vi "Combustion Setup 1.vi"() -> ()   [LabVIEW 2018]
doc: "Simplified example program for initializing the COM port, determining the data frame of an Alicat, acquiring the data of the same Alicat, and writing a setpoint to the same device. \n\nThis is a slightly more feature rich version of the Alicat Simplified Driver Example, and contains an example of a method for easily implementing fast setpoint writes."
panel:
  in  "Stopping Flow Rate (Top)":dbl format="%_4g"
  in  "Initial Flow Rate (Top)":dbl format="%_4g"
  in  "Top COM Port Settings (always Unit ID = B; methane)":T1={"Unit ID"="A", "Baud Rate"=enum."19200", "VISA Sesssion In"="COM1"}
  in  "Stopping Flow Rate (Bottom)":dbl format="%_4g"
  in  "Stop Running Button":bool
  in  "Initial Flow Rate (Bottom)":dbl format="%_4g"
  in  "Bottom COM Port Settings (always Unit ID = A; oxygen)":T1={"Unit ID"="A", "Baud Rate"=enum."19200", "VISA Sesssion In"="COM1"}
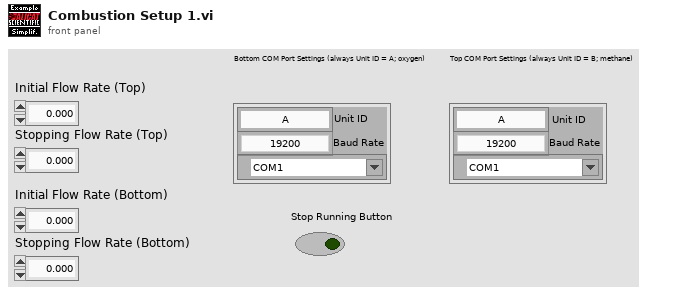
[diagram p1: front panel]
types:
  T1 = cluster{"Unit ID":string, "Baud Rate":enum8{"2400", "9600", "19200", "38400", "57600", "115200", "Unknown"}, "VISA Sesssion In":refnum<visa-resource-name>}
  T2 = cluster{"Absolute Pressure":bool, "Gauge/Diff. Pressure":bool, "Barometric Pressure":bool, "Temperature":bool, "Volumetric":bool, "Mass":bool, "Setpoint":bool, "Valve Drive":bool, "Totalizer":bool, "Totalizer Timer":bool, "Totalizer Average Flow":bool, "Totalizer Peak Flow":bool, "Gas Selected":bool, "Tot. Timer Format":u16}
  T3 = cluster{"Controller Full Scale":dbl, "Controller Select":u16, "Control Range":enum16{"Normal", "Inverted", "Bidirectional", "Unknown"}}
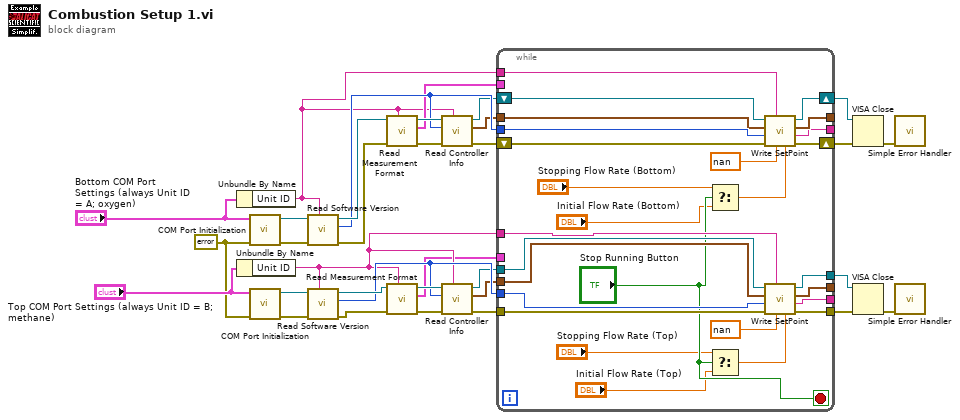
[diagram p0: block diagram]
diagram:
  w1 = errorcluster {"status"=FALSE, "code"=0, "source"=""} ("error in (no error)")
  n1 = Unbundle By Name("Bottom COM Port Settings (always Unit ID = A; oxygen)") -> ("Unit ID"=w6:string)
  n2 = Unbundle By Name("Top COM Port Settings (always Unit ID = B; methane)") -> ("Unit ID"=w17:string)
  n3 = call "COM Port Initialization.vi"("error in (no error)"=w1, "Communication Settings"="Bottom COM Port Settings (always Unit ID = A; oxygen)") -> ("error out"=w4:errorcluster, "VISA Session Out"=w3:refnum<visa-resource-name>)  [unwired: 8 in]
  n4 = call "COM Port Initialization.vi"("error in (no error)"=w1, "Communication Settings"="Top COM Port Settings (always Unit ID = B; methane)") -> ("error out"=w8:errorcluster, "VISA Session Out"=w9:refnum<visa-resource-name>)  [unwired: 8 in]
  n5 = call "Read Software Version.vi"("Unit ID (A)"=w6, "error in"=w4, "VISA Session In"=w3) -> ("error out"=w31:errorcluster, "Software Version"=w29:u8, "VISA Session Out"=w30:refnum<visa-resource-name>)  [unwired: 6 in]
  n6 = call "Read Software Version.vi"("Unit ID (A)"=w17, "error in"=w8, "VISA Session In"=w9) -> ("error out"=w22:errorcluster, "Software Version"=w20:u8, "VISA Session Out"=w21:refnum<visa-resource-name>)  [unwired: 6 in]
  n7 = call "Read Measurement Format.vi"("Unit ID (A)"=w6, "error in"=w31, "VISA Session In"=w30) -> ("error out"=w33:errorcluster, "Data Frame Format"=w7:T2, "VISA Session Out"=w32:refnum<visa-resource-name>)  [unwired: 6 in]
  n8 = call "Read Measurement Format.vi"("Unit ID (A)"=w17, "error in"=w22, "VISA Session In"=w21) -> ("error out"=w24:errorcluster, "Data Frame Format"=w5:T2, "VISA Session Out"=w23:refnum<visa-resource-name>)  [unwired: 6 in]
  n9 = call "Read Controller Info.vi"("Unit ID (A)"=w6, "error in"=w33, "Software Version"=w29, "VISA Session In"=w32) -> ("error out"=w28:errorcluster, "Controller Info out"=w27:T3, "VISA Session Out"=w26:refnum<visa-resource-name>)  [unwired: 4 in, 1 out]
  n10 = call "Read Controller Info.vi"("Unit ID (A)"=w17, "error in"=w24, "Software Version"=w20, "VISA Session In"=w23) -> ("error out"=w19:errorcluster, "Controller Info out"=w18:T3, "VISA Session Out"=w16:refnum<visa-resource-name>)  [unwired: 4 in, 1 out]
  n11 = while {
    tunnel: w29 -> [w60]
    tunnel: w27 -> [w58]
    tunnel: w20 -> [w54]
    tunnel: w19 -> [w53]
    tunnel: w18 -> [w52]
    tunnel: w17 -> [w51]
    tunnel: w16 -> [w49]
    shift-right: [w46] -> w14
    shift-left: w28 -> [w59]
    shift-right: [w47] -> w15
    shift-left: w26 -> [w56]
    tunnel: [w44] -> w12
    tunnel: [w43] -> w11
    tunnel: [w42] -> _
    tunnel: [w41] -> _
    tunnel: [w40] -> _
    tunnel: [w39] -> _
    tunnel: w7 -> [_]
    tunnel: w6 -> [w38]
    tunnel: w5 -> [_]
    stop <- "Stop Running Button" stop-if-true
    n12 = Select(t="Stopping Flow Rate (Bottom)", s="Stop Running Button", f="Initial Flow Rate (Bottom)") -> (s? t:f=w55:dbl)
    n13 = Select(t="Stopping Flow Rate (Top)", s="Stop Running Button", f="Initial Flow Rate (Top)") -> (s? t:f=w48:dbl)
    n14 = call "Write SetPoint.vi"("Setpoint"=w55, "Previous Setpoint"=nan ("Setpoint"), "Unit ID (A)"=w38, "error in"=w59, "Software Version"=w60, "Controller Info out"=w58, "VISA Session In"=w56) -> ("error out"=w46:errorcluster, "Data frame returned"=w41:string, "Controller Info out"=w42:T3, "VISA Session Out"=w47:refnum<visa-resource-name>)  [unwired: 1 in]
    n15 = call "Write SetPoint.vi"("Setpoint"=w48, "Previous Setpoint"=nan ("Setpoint"), "Unit ID (A)"=w51, "error in"=w53, "Software Version"=w54, "Controller Info out"=w52, "VISA Session In"=w49) -> ("error out"=w43:errorcluster, "Data frame returned"=w39:string, "Controller Info out"=w40:T3, "VISA Session Out"=w44:refnum<visa-resource-name>)  [unwired: 1 in]
  }
  n16 = VISA Close(VISA resource name=w15, error in (no error)=w14) -> (error out=w25:errorcluster)
  n17 = VISA Close(VISA resource name=w12, error in (no error)=w11) -> (error out=w13:errorcluster)
  n18 = call <vilib>:"Simple Error Handler.vi"("error in (no error)"=w25) -> ()  [unwired: 4 in, 5 out]
  n19 = call <vilib>:"Simple Error Handler.vi"("error in (no error)"=w13) -> ()  [unwired: 4 in, 5 out]
